vi "Switch Notifier.vi"(8 "error in (no error)":errorcluster, 10 "Station":i32, 11 "All Display Notifiers":T1) -> (0 "error out":errorcluster, 3 "Notifier Out":refnum<queue>)   [LabVIEW 2014]
uses:
  All Display Notifiers.ctl
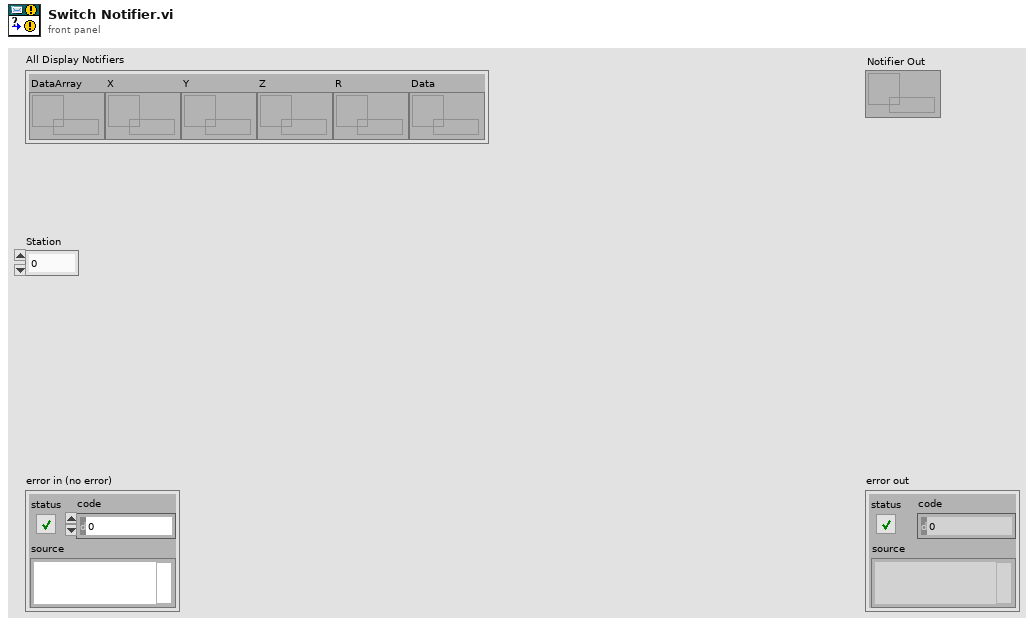
[diagram p1: front panel]
types:
  T1 = typedef "All Display Notifiers.ctl" = cluster{"DataArray":refnum<queue>, "X":refnum<queue>, "Y":refnum<queue>, "Z":refnum<queue>, "R":refnum<queue>, "Data":refnum<queue>}
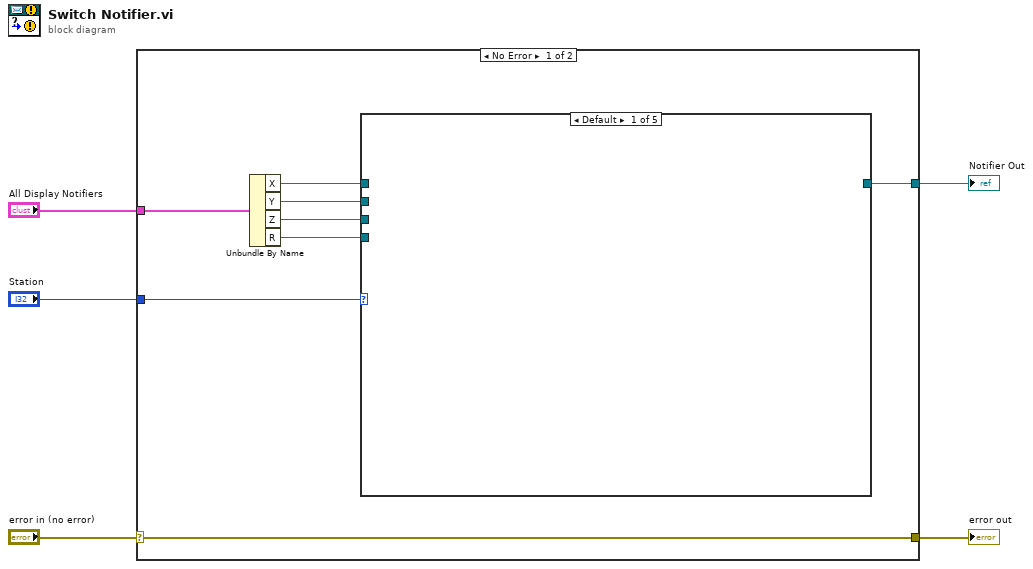
[diagram p0: block diagram]
diagram:
  n1 = case shown="No Error" "error in (no error)" {
    selector: "error in (no error)" -> [w6 w18]
    tunnel: "Station" -> [w13 _]
    tunnel: "All Display Notifiers" -> [w12 _]
    tunnel: [w7 _] -> w1
    tunnel: [w6 w18] -> w2
    frame No Error {
      n2 = Unbundle By Name(w12) -> ("X"=w11:refnum<queue>, "Y"=w10:refnum<queue>, "Z"=w9:refnum<queue>, "R"=w8:refnum<queue>)
      n3 = case shown="Default" w13 {
        tunnel: w11 -> [_ w14 _ _ _]
        tunnel: w10 -> [_ _ w15 _ _]
        tunnel: w9 -> [_ _ _ w16 _]
        tunnel: w8 -> [_ _ _ _ w17]
        tunnel: [_ w14 w15 w16 w17] -> w7
        frame Default {
        }
        frame 1 {
        }
        frame 2 {
        }
        frame 3 {
        }
        frame 4 {
        }
      }
    }
    frame Error {
    }
  }
  "error out" <- w2
  "Notifier Out" <- w1
